vi "Mask TF Chart.vi"(1 "Mask Array":bool[][](array[boolean]), 2 "TF plot":u8[][](array[numeric])) -> (0 "TF plot Out":u8[][](array[numeric]))   [LabVIEW 2017]
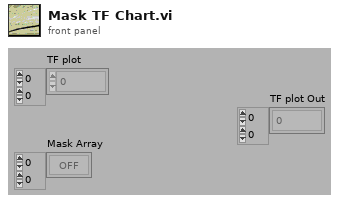
[diagram p1: front panel]
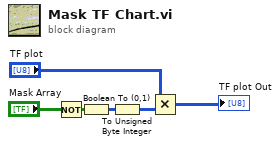
[diagram p0: block diagram]
diagram:
  n1 = Not(x="Mask Array") -> (.not. x?=w4:bool[][])
  n2 = Boolean To (0,1)(Boolean=w4) -> (0, 1=w3:i16[][])
  n3 = To Unsigned Byte Integer(number=w3) -> (unsigned 8bit integer=w2:u8[][])
  n4 = Multiply(x="TF plot", y=w2) -> (x*y=→"TF plot Out":u8[][])
